vi "output_type.vi"() -> ()   [LabVIEW 2017]
panel:
  out "添加的数组 2":bool[](array[boolean])=[TRUE, FALSE, TRUE]
  out "数字":u32=5 format="%x"
  out "添加的数组":bool[](array[boolean])=[TRUE, FALSE, TRUE]
  in  "clkout":bool
  in  "Calib":bool
  in  "TiriggerID":bool
  in  "address":string="192.168.10.34"
  in  "error in (no error)":errorcluster
  out "error out":errorcluster
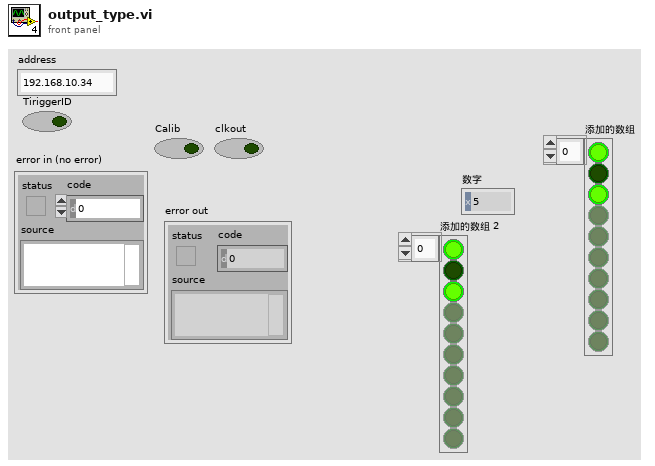
[diagram p1: front panel]
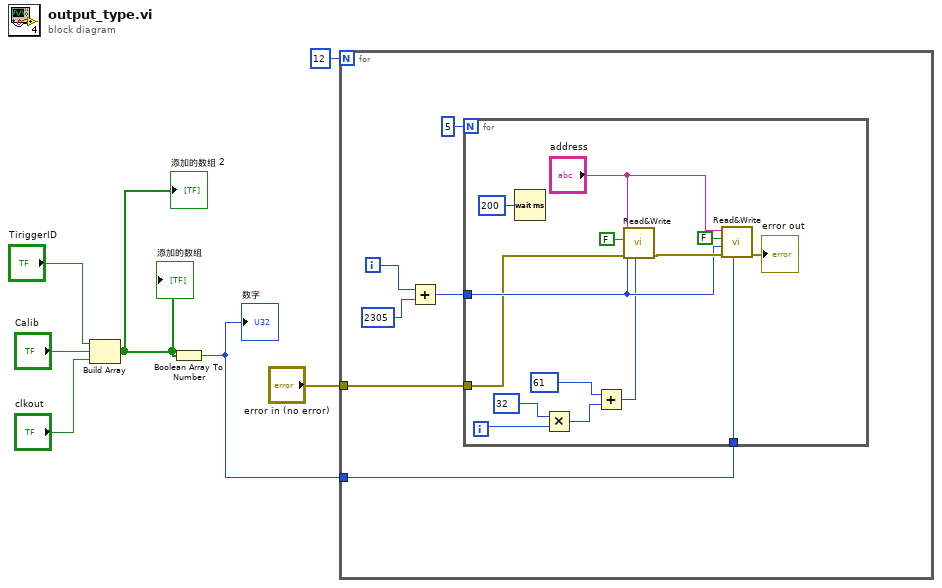
[diagram p0: block diagram]
diagram:
  n1 = Build Array("TiriggerID", "Calib", "clkout") -> (w3:bool[])
  "添加的数组" <- w3
  "添加的数组 2" <- w3
  n2 = Boolean Array To Number(Boolean array=w3) -> (number=w4:u32)
  "数字" <- w4
  n3 = for {
    N: 12 -> [_]
    tunnel: w4 -> [w13]
    tunnel: "error in (no error)" -> [w8]
    i -> [w10]
    n4 = Add(x=w10, y=u32 2305 ("Address")) -> (x+y=w11:u32)
    n5 = for {
      N: 5 -> [_]
      tunnel: w13 -> [w22]
      tunnel: w11 -> [w21]
      tunnel: w8 -> [w15]
      i -> [w19]
      n6 = Wait (ms)(milliseconds to wait=u32 200 ("等待时间（毫秒）")) -> ()  [unwired: 1 out]
      n7 = Multiply(x=u8 32 ("In"), y=w19) -> (x*y=w17:i32)
      n8 = Add(x=u8 61 ("In"), y=w17) -> (x+y=w16:i32)
      n9 = call "Read&Write.vi"("In"=w16, "error in (no error)"=w15, "Address"=w21, "Read (TRUE)"=FALSE, "address"="address") -> ("error out"=w27:errorcluster)  [unwired: 5 in, 1 out]
      n10 = call "Read&Write.vi"("In"=w22, "error in (no error)"=w27, "Address"=w21, "Read (TRUE)"=FALSE, "address"="address") -> ("error out"=→"error out":errorcluster)  [unwired: 5 in, 1 out]
    }
  }
